vi "CRYGet Post P Array.vi"() -> (1 "PP Wave Array":T1(array[cluster]), 2 "PP Value Array":T1(array[cluster]), 3 "PP Curve Array":T1(array[cluster]))   [LabVIEW 2013]
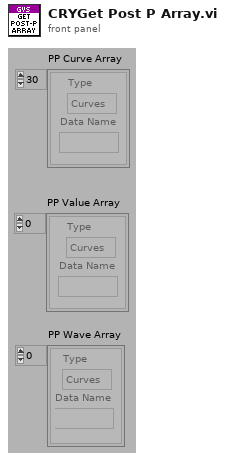
[diagram p1: front panel]
types:
  T1 = cluster{"Type":enum16{"Curves", "Values", "Results", "WFM"}, "Data Name":string}[]
  T2 = cluster{"CurveTabName":u16, "Operand Name":string}
  T3 = cluster{"CurveTabName":u16, "Operand Name":string}[]
  T4 = typedef "CRYData Cluster.ctl" = cluster{"Name":string, "Curve":cluster{"x":dbl, "y":dbl, "z":dbl}[], "X data":u16, "Y data":u16, "Z data":u16, "X axis":u16, "Y axis":u16, "Z axis":u16, "X unit":string, "Y unit":string, "Z unit":string, "X dB ref":dbl, "Y dB ref":dbl, "Z dB ref":dbl, "single val":bool, "protected":bool, "display X":bool, "display Y":bool, "display Z":bool, "Test Info":string, "Step No.":i32, "Plot Settings":cluster{"Color":u32, "Interpolation":u8, "Point Style":u8, "Line Style":u8, "Point Color":u32, "Line Width":u8, "Bar Plot Style":u8, "Fill To":i16}, "AutoProtect":bool}
  T5 = typedef "CRYWaveform Cluster.ctl" = cluster{"Waveform":cluster{"X0":dbl, "dX":dbl, "Y":sgl[]}, "X data":u16, "Y data":u16, "Y axis":u16, "X unit":string, "Y unit":string, "Y dB ref":dbl, "display Y":bool, "display X":bool, "Overload?":bool, "Test Info":string, "Step No.":i32, "Name":string, "protected":bool, "Sqc history":string[], "Signal Channel ID":i32, "Plot Settings":cluster{"Color":u32, "Interpolation":u8, "Point Style":u8, "Line Style":u8, "Point Color":u32, "Line Width":u8, "Bar Plot Style":u8, "Fill To":i16}, "AutoProtect":bool}
  T6 = cluster{"Type":enum16{"Curves", "Values", "Results", "WFM"}, "Name":string}
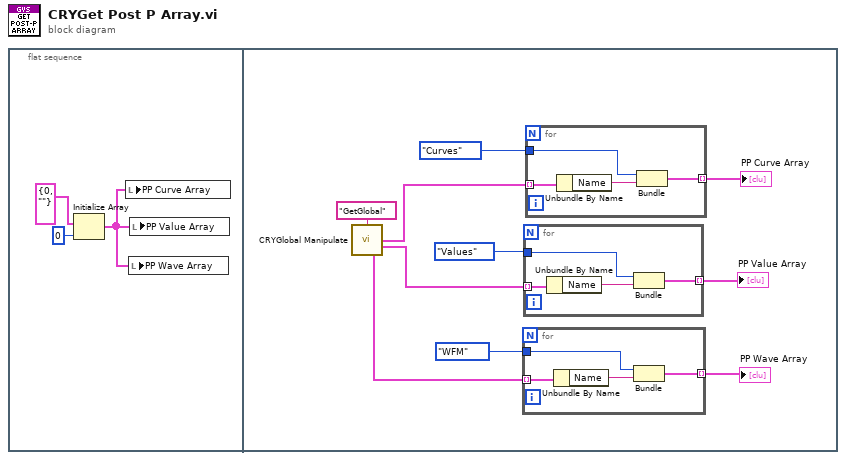
[diagram p0: block diagram]
diagram:
  n1 = flat-sequence {
    frame #0 {
      n2 = Initialize Array(T2 {"CurveTabName"=0, "Operand Name"=""} ("element"), 0 ("dimension size")) -> (w1:T3)
      n3 = local write "PP Curve Array"(w1) -> ()
      n4 = local write "PP Wave Array"(w1) -> ()
      n5 = local write "PP Value Array"(w1) -> ()
    }
    frame #1 {
      n6 = call "CRYGlobal Manipulate.vi"("sAction"="GetGlobal") -> ("Curves Out"=w6:T4[], "Values Out"=w5:T4[], "WFM Out"=w4:T5[])  [unwired: 8 in, 4 out]
      n7 = for {
        tunnel: w4 -> [w21] mode=indexing
        tunnel: enum16{"Curves", "Values", "Results", "WFM"}."WFM" ("Type") -> [w20]
        tunnel: [w18] -> w13 mode=indexing
        n8 = Unbundle By Name(w21) -> ("Name"=w19:string)
        n9 = Bundle("Type"=w20, "Name"=w19) -> (w18:T6)  [unwired: 1 out]
      }
      "PP Wave Array" <- w13
      n10 = for {
        tunnel: w5 -> [w17] mode=indexing
        tunnel: enum16{"Curves", "Values", "Results", "WFM"}."Values" ("Type") -> [w15]
        tunnel: [w14] -> w8 mode=indexing
        n11 = Unbundle By Name(w17) -> ("Name"=w16:string)
        n12 = Bundle("Type"=w15, "Name"=w16) -> (w14:T6)  [unwired: 1 out]
      }
      "PP Value Array" <- w8
      n13 = for {
        tunnel: w6 -> [w24] mode=indexing
        tunnel: enum16{"Curves", "Values", "Results", "WFM"}."Curves" ("Type") -> [w25]
        tunnel: [w22] -> w9 mode=indexing
        n14 = Unbundle By Name(w24) -> ("Name"=w23:string)
        n15 = Bundle("Type"=w25, "Name"=w23) -> (w22:T6)  [unwired: 1 out]
      }
      "PP Curve Array" <- w9
    }
  }
